vi "ApplicationGlobal.vi"() -> ()   [LabVIEW 2016]
uses:
  tools/Windows/Windows.ExitAction.ctl
panel:
  in  "VariantsFolder":path=path "C:/Private/ProdaCommunicationStation/SOFTWARE/logs/tmp/variants"
  in  "ExportedPath":path=path "C:/Private/ProdaCommunicationStation/SOFTWARE/logs/tmp/exported"
  in  "ArchivedPath":path=path "C:/Private/ProdaCommunicationStation/SOFTWARE/logs/tmp/arch"
  out "Stats.Prog%":dbl format="%.3f"
  out "DMCConfig.Unlock":bool
  out "Runtime":bool
  out "AppLaunched":bool
  in  "EventPath":path=path "D:/Maszup/WABCO/SVN/LaserMarkingStation/SOFTWARE/logs/events"
  in  "ResultPath":path=path "C:/Private/ProdaCommunicationStation/SOFTWARE/logs/tmp"
  out "AppDate":string
  in  "Status":string
  in  "ExitAction":T1=enum."Shut Down PC"
  out "AppName":string
  out "Changelog":string
  out "AppVer":string
  out "Quitting":bool
  in  "LogPath":path=path "D:/Maszup/WABCO/SVN/LaserMarkingStation/SOFTWARE/logs"
  in  "SettingsPath":path=path "D:/Maszup/WABCO/SVN/LaserMarkingStation/SOFTWARE/settings"
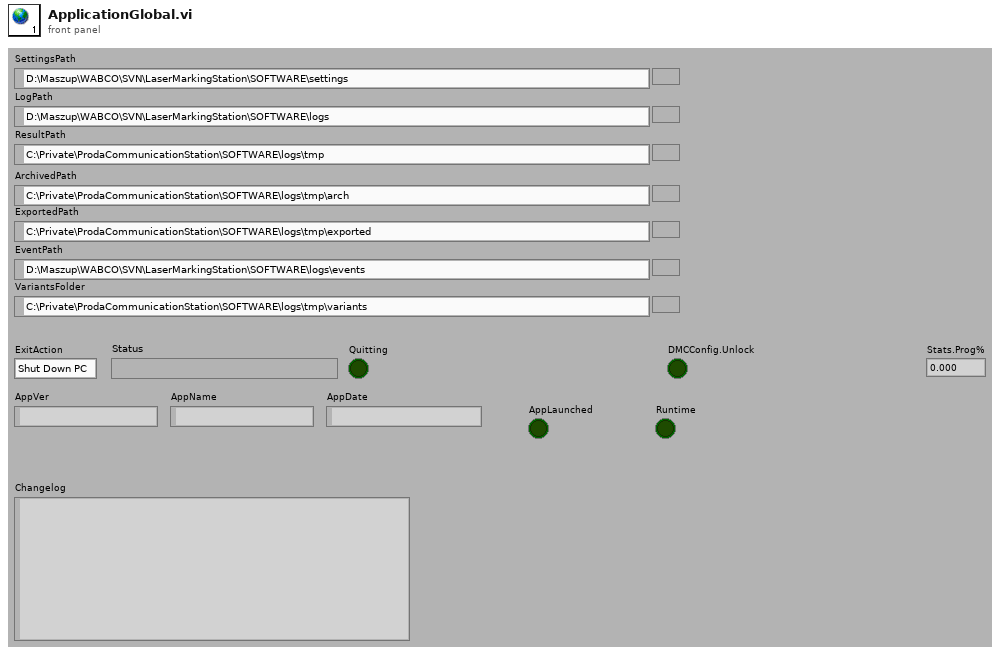
[diagram p1: front panel]
types:
  T1 = typedef "Windows.ExitAction.ctl" = enum16{"Log off from PC", "Shut Down PC", "Reboot PC", "Close Program"}
diagram:
